vi "Mean (CDB).vi"(0 "X":cdb[](array[numeric])) -> (1 "mean":cdb, 2 "error":i32)   [LabVIEW 2014, in "NI_AALBase.lvlib"]
doc: "Computes the <B>mean</B> of the values in the input sequence <B>X</B>. You must manually select the polymorphic instance you want to use."
uses:
  NI_AALBase.lvlib
panel:
  # "Complex Mean"
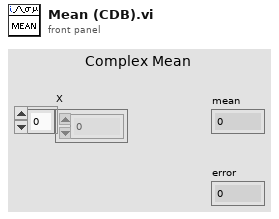
[diagram p1: front panel]
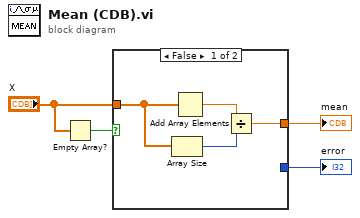
[diagram p0: block diagram]
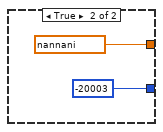
[diagram p2: hidden frame]
diagram:
  n1 = Empty Array?(array="X") -> (empty?=w4:bool)
  n2 = case shown="False" w4 {
    tunnel: "X" -> [w8 _]
    tunnel: [w5 cdb nan+nani] -> w2
    tunnel: [_ -20003] -> w1
    frame False {
      n3 = Array Size(array=w8) -> (size(s)=w6:i32)
      n4 = Add Array Elements(numeric array=w8) -> (sum=w7:cdb)
      n5 = Divide(x=w7, y=w6) -> (x/y=w5:cdb)
    }
    frame True {
    }
  }
  "mean" <- w2
  "error" <- w1
